vi "AlliGator Save Phasor Plot Additional Data.vi"(4 "Save only if selected":bool, 6 "Save as...":bool, 7 "Phasor Plot Folder Path (empty)":path, 8 "error in (no error)":errorcluster, 9 "Raw Phasor Plot":T1={"Phasor Plot Name"="", "Raw Phasor Plot"=[], "Phasor Frequency"=160000000.0, "[Decay Metadata]"=[], "Raw Phasor Plot SDV"=[], "Phasor SDV Options"={"Compute Estimated SDV"=FALSE, "# Replicas"=100, "Use Estimated Average Phasor"=FALSE}, "[Calibration Phasor]"=[]} {"[Decay Metadata]"."# Folds" min=1; "[Decay Metadata]"."ROI Descriptor"."Contours"."Type" items=["No Selection", "Point", "Line", "Rectangle", "Oval", "Polygon", "Freehand Region", "Annulus", "Unused2", "Unused3", "Broken Line", "Freehand Line", "Rotated Rectangle"]}, 10 "Selected Plot":i32, 11 "Phasor Graph":refnum<vi>) -> (0 "Error Out":errorcluster, 1 "Message":string)   [LabVIEW 2021, in "AlliGator Phasor Graph.lvlib"]
doc: "Save the user-selected Phasor Plot additional data."
uses:
  AlliGator Phasor Graph.lvlib
  AlliGator Raw Phasor Plot Data v4.ctl
  Phasor/Phasor (g, s).ctl
  AlliGator Decay Metadata v3.ctl
  AlliGator Decay Background Subtraction Info.ctl
  AlliGator Baseline Subtraction Method.ctl
  Graphs/XY Graph/XY Graph Plot Shift Parameters.ctl
  Graphs/XY Graph/XY Graph Plot Shift Method.ctl
  AlliGator Decay Extrapolation Parameters.ctl
  Phasor/Phasor Standard Deviation Options.ctl
  Phasor/Calibration Phasor (m, phi).ctl
  Phasor/Phasor.lvlib
  AlliGator Decay Preprocessing.lvlib
  Graphs/XY Graph/XY Graph Add-Ons.lvlib
panel:
  # "see the AlliGator License on the block diagram (Ctrl+E or Window:Show Block Diagram)"
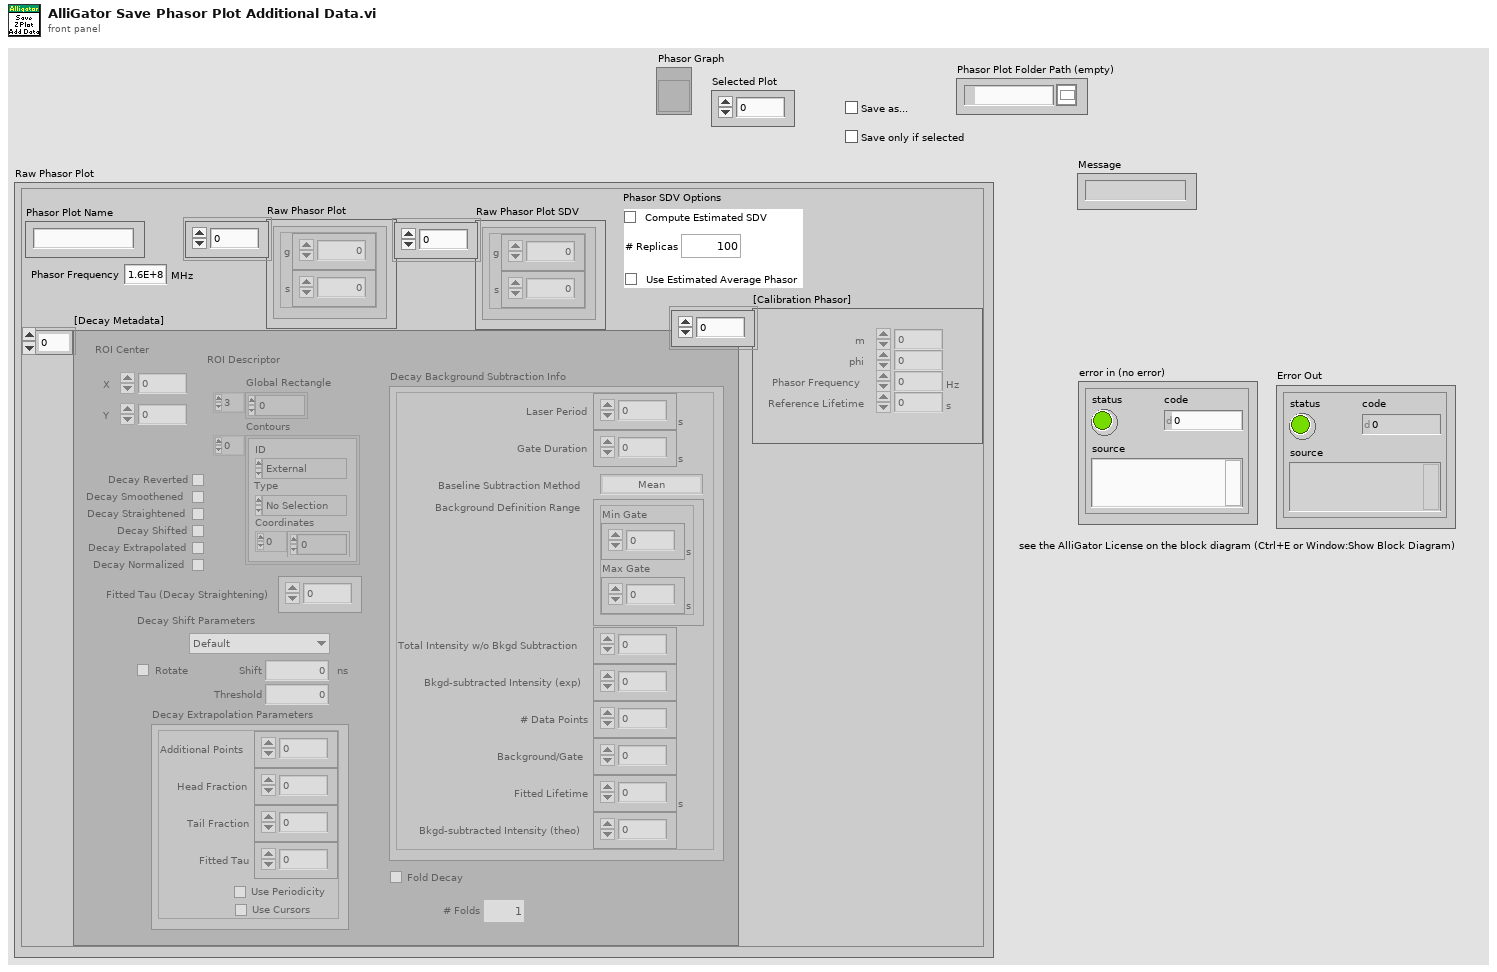
[diagram p1: front panel]
types:
  T1 = typedef "AlliGator Phasor Graph.lvlib/AlliGator Raw Phasor Plot Data v4.ctl" = cluster{"Phasor Plot Name":string, "Raw Phasor Plot":T2[], "Phasor Frequency":dbl[unit], "[Decay Metadata]":T3[], "Raw Phasor Plot SDV":T2[], "Phasor SDV Options":T10, "[Calibration Phasor]":T11[]}
  T2 = typedef "Phasor.lvlib/Phasor (g, s).ctl" = cluster{"g":dbl, "s":dbl}
  T3 = typedef "AlliGator Phasor Graph.lvlib/AlliGator Decay Metadata v3.ctl" = cluster{"ROI Descriptor":T4, "ROI Center":cluster{"X":i32, "Y":i32}, "Decay Background Subtraction Info":T5, "Decay Reverted":bool, "Decay Smoothened":bool, "Decay Straightened":bool, "Fitted Tau (Decay Straightening)":dbl, "Decay Shift Parameters":T7, "Decay Shifted":bool, "Decay Extrapolated":bool, "Decay Extrapolation Parameters":T9, "Decay Normalized":bool, "Fold Decay":bool, "# Folds":u32}
  T4 = typedef "ROI Descriptor" = cluster{"Global Rectangle":i32[], "Contours":cluster{"ID":enum32{"External", "Internal"}, "Type":u32, "Coordinates":i32[]}[]}
  T5 = typedef "AlliGator Decay Analysis.lvlib/AlliGator Decay Preprocessing.lvlib/AlliGator Decay Background Subtraction Info.ctl" = cluster{"Laser Period":dbl[unit], "Gate Duration":dbl[unit], "Baseline Subtraction Method":T6, "Background Definition Range":cluster{"Min Gate":dbl[unit], "Max Gate":dbl[unit]}, "Total Intensity w/o Bkgd Subtraction":dbl, "Bkgd-subtracted Intensity (exp)":dbl, "# Data Points":i32, "Background/Gate":dbl, "Fitted Lifetime":dbl[unit], "Bkgd-subtracted Intensity (theo)":dbl}
  T6 = typedef "AlliGator Decay Analysis.lvlib/AlliGator Decay Preprocessing.lvlib/AlliGator Baseline Subtraction Method.ctl" = enum16{"Mean", "Min", "Square Gated Single-Exponential", "File", "Constant"}
  T7 = typedef "XY Graph Add-Ons.lvlib/XY Graph Plot Shift Parameters.ctl" = cluster{"Type":T8, "Shift":dbl[unit], "Threshold":dbl, "Rotate":bool}
  T8 = typedef "XY Graph Add-Ons.lvlib/XY Graph Plot Shift Method.ctl" = enum16{"Default", "CFD", "Threshold", "Cross-Correlation"}
  T9 = typedef "AlliGator Decay Analysis.lvlib/AlliGator Decay Preprocessing.lvlib/AlliGator Decay Extrapolation Parameters.ctl" = cluster{"Additional Points":u32, "Head Fraction":dbl, "Fitted Tau":dbl, "Use Periodicity":bool, "Use Cursors":bool, "Tail Fraction":dbl}
  T10 = typedef "Phasor.lvlib/Phasor Standard Deviation Options.ctl" = cluster{"Compute Estimated SDV":bool, "# Replicas":u32, "Use Estimated Average Phasor":bool}
  T11 = typedef "Phasor.lvlib/Calibration Phasor (m, phi).ctl" = cluster{"m":dbl, "phi":dbl, "Phasor Frequency":dbl[unit], "Reference Lifetime":dbl[unit]}
  T12 = typedef "AlliGator Phasor Graph.lvlib/AlliGator Phasor Plot Exported Data Selection.ctl" = cluster{"x":bool, "y":bool, "g":bool, "s":bool, "phi":bool, "m":bool, "tau phi":bool, "tau m":bool, "phasor ratio (intensity-weighted)":bool, "<tau> (intensity-weighted)":bool, "phasor ratio (amplitude-weighted)":bool, "<tau> (amplitude-weighted)":bool, "g SDV":bool, "s SDV":bool, "phi SDV":bool, "m SDV":bool, "tau phi SDV":bool, "tau m SDV":bool, "phasor ratio (intensity-weighted) SDV":bool, "<tau> (intensity-weighted) SDV":bool, "phasor ratio (amplitude-weighted) SDV":bool, "<tau> (amplitude-weighted) SDV":bool}
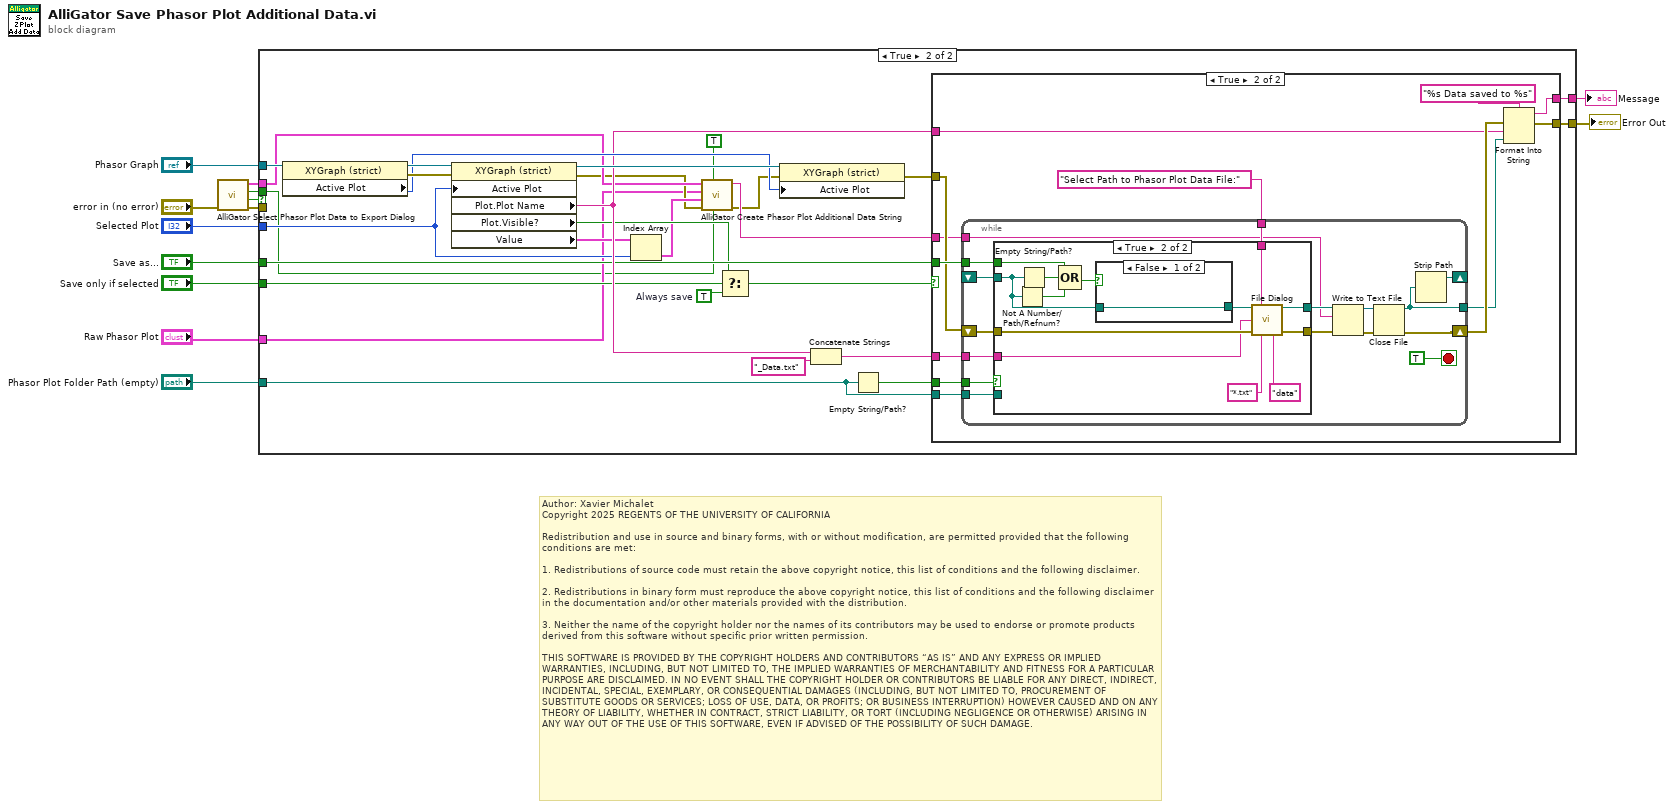
[diagram p0: block diagram]
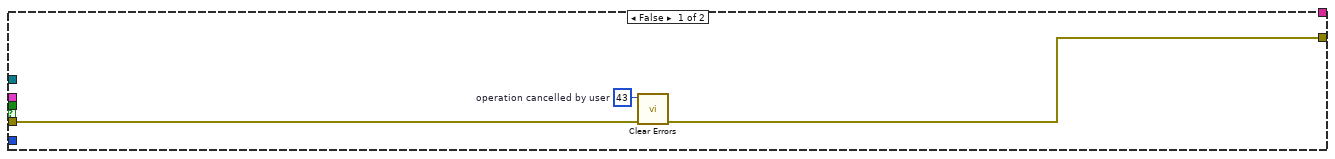
[diagram p2: hidden frame]
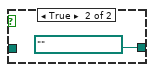
[diagram p5: hidden frame]
diagram:
  # "Author: Xavier Michalet\nCopyright 2025 REGENTS OF THE UNIVERSITY OF CALIFORNIA\n\nRedistribution and use in source and binary forms, with or without modification, are permitted provided that the following conditions are met:\n\n1. Redistributions of source code must retain the above copyright notice, this list of conditions and the following disclaimer.\n\n2. Redistributions in binary form must reproduce the above copyright notice, this list of conditions and the following disclaimer in the documentation and/or other materials provided with the distribution.\n\n3. Neither the name of the copyright holder nor the names of its contributors may be used to endorse or promote products derived from this software without specific prior written permission.\n\nTHIS SOFTWARE IS PROVIDED BY THE COPYRIGHT HOLDERS AND CONTRIBUTORS “AS IS” AND ANY EXPRESS OR IMPLIED WARRANTIES, INCLUDING, BUT NOT LIMITED TO, THE IMPLIED WARRANTIES OF MERCHANTABILITY AND FITNESS FOR A PARTICULAR PURPOSE ARE DISCLAIMED. IN NO EVENT SHALL THE COPYRIGHT HOLDER OR CONTRIBUTORS BE LIABLE FOR ANY DIRECT, INDIRECT, INCIDENTAL, SPECIAL, EXEMPLARY, OR CONSEQUENTIAL DAMAGES (INCLUDING, BUT NOT LIMITED TO, PROCUREMENT OF SUBSTITUTE GOODS OR SERVICES; LOSS OF USE, DATA, OR PROFITS; OR BUSINESS INTERRUPTION) HOWEVER CAUSED AND ON ANY THEORY OF LIABILITY, WHETHER IN CONTRACT, STRICT LIABILITY, OR TORT (INCLUDING NEGLIGENCE OR OTHERWISE) ARISING IN ANY WAY OUT OF THE USE OF THIS SOFTWARE, EVEN IF ADVISED OF THE POSSIBILITY OF SUCH DAMAGE."
  n1 = call "AlliGator Select Phasor Plot Data to Export Dialog.vi"("error in (no error)"="error in (no error)") -> ("error out"=w5:errorcluster, "OK?"=w4:bool, "Average Plot Data"=w2:bool, "Phasor Plot Exported Data"=w3:T12)  [unwired: 7 in]
  n2 = case shown="True" w4 {
    tunnel: "Phasor Graph" -> [_ w44]
    tunnel: "Selected Plot" -> [_ w24]
    tunnel: [w15 w39] -> w11
    tunnel: "Raw Phasor Plot" -> [_ w20]
    tunnel: "Save as..." -> [_ w34]
    tunnel: "Phasor Plot Folder Path (empty)" -> [_ w32]
    tunnel: "Save only if selected" -> [_ w31]
    tunnel: w5 -> [w16 _]
    tunnel: w3 -> [_ w26]
    tunnel: w2 -> [_ w19]
    tunnel: [_ w17] -> w1
    frame False {
      w14 = 43  # operation cancelled by user
      n3 = call <vilib>:"Clear Errors.vi"("error in (no error)"=w16, "specific error code to clear (0: all)"=w14) -> ("error out"=w15:errorcluster)  [unwired: 4 in, 1 out]
    }
    frame True {
      w30 = TRUE  # Always save
      n4 = property class="XYGraph (strict)"(reference=w44) -> (reference out=w43:refnum<vi>, error out=w42:errorcluster, "Active Plot"=w40:u32)  [unwired: 1 in]
      n5 = property class="XYGraph (strict)"(reference=w43, error in=w42, "Active Plot"=w24) -> (reference out=w41:refnum<vi>, error out=w22:errorcluster, "Plot.Plot Name"=w38:string, "Plot.Visible?"=w29:bool, "Value"=w25:cluster{dbl[], dbl[]}[])
      n6 = Index Array(array=w25, index=w24) -> (element=w23:cluster{dbl[], dbl[]})
      n7 = call "AlliGator Create Phasor Plot Additional Data String.vi"("Average Plot Data (F)"=w19, "Include Header String (F)"=TRUE ("Include Headre  String"), "error in (no error)"=w22, "Calibrated Phasor Plot"=w23, "Raw Phasor Plot"=w20, "Phasor Plot Exported Data"=w26) -> ("error out"=w21:errorcluster, "Phasor Plot Additional Data String"=w27:string)  [unwired: 4 in]
      n8 = Select(t=w29, s=w31, f=w30) -> (s? t:f=w28:bool)
      n9 = property class="XYGraph (strict)"(reference=w41, error in=w21, "Active Plot"=w40) -> (error out=w35:errorcluster)  [unwired: 1 out]
      n10 = Concatenate Strings(w38, "_Data.txt" ("string")) -> (w36:string)
      n11 = Empty String/Path?(string/path=w32) -> (empty?=w33:bool)
      n12 = case shown="True" w28 {
        tunnel: [w45 w46] -> w39
        tunnel: w38 -> [_ w55]
        tunnel: w36 -> [_ w53]
        tunnel: w35 -> [w45 w49]
        tunnel: w34 -> [_ w52]
        tunnel: w33 -> [_ w51]
        tunnel: w32 -> [_ w50]
        tunnel: w27 -> [_ w48]
        tunnel: [_ w47] -> w17
        frame False {
        }
        frame True {
          n13 = while {
            tunnel: w48 -> [w65]
            tunnel: [w61] -> w56
            shift-right: [w62] -> w57
            shift-left: w49 -> [w69]
            shift-right: [w74] -> _
            shift-left: _ -> [w71]
            tunnel: w52 -> [w72]
            tunnel: "Select Path to Phasor Plot Data File:" ("Prompt") -> [w70]
            tunnel: w53 -> [w68]
            tunnel: w51 -> [w60]
            tunnel: w50 -> [w59]
            stop <- TRUE stop-if-true
            n14 = case shown="True" w60 {
              tunnel: w72 -> [_ w87]
              tunnel: w71 -> [_ w85]
              tunnel: w70 -> [_ w83]
              tunnel: w69 -> [w75 w82]
              tunnel: w68 -> [_ w79]
              tunnel: [w76 w78] -> w67
              tunnel: [w75 w77] -> w66
              tunnel: w59 -> [w76 _]
              frame False {
              }
              frame True {
                n15 = Not A Number/Path/Refnum?(number/path/refnum=w85) -> (NaN/Path/Refnum?=w88:bool)
                n16 = Empty String/Path?(string/path=w85) -> (empty?=w89:bool)
                n17 = Compound Arithmetic op=OR(w87, w89, w88) -> (w86:bool)
                n18 = case shown="False" w86 {
                  tunnel: [w90 path "" ("start path  (Not A Path)")] -> w84
                  tunnel: w85 -> [w90 _]
                  frame False {
                  }
                  frame True {
                  }
                }
                n19 = call "File Dialog"("start path"=w84, "prompt"=w83, "default name"=w79, "error in"=w82, "pattern (all files)"="*.txt" ("Pattern (*.xml;*.XML)"), "pattern label"="data" ("File Extension (xml)")) -> ("selected path"=w78:path, "error out"=w77:errorcluster)  [unwired: 6 in, 2 out]
              }
            }
            n20 = Write to Text File(file (use dialog)=w67, text=w65, error in=w66) -> (refnum out=w64:refnum<file>, error out=w63:errorcluster)  [unwired: 1 in, 1 out]
            n21 = Close File(refnum=w64, error in=w63) -> (path=w61:path, error out=w62:errorcluster)
            n22 = Strip Path(path=w61) -> (stripped path=w74:path)  [unwired: 1 out]
          }
          n23 = Format Into String(format string="%s Data saved to %s", error in=w57, w55, w56) -> (resulting string=w47:string, error out=w46:errorcluster)  [unwired: 1 in]
        }
      }
    }
  }
  "Error Out" <- w11
  "Message" <- w1
